vi "connect.vi"(8 "error in (no error)":errorcluster, 11 "TCPClient in":refnum<class "TCPClient.lvclass">) -> (0 "error out":errorcluster, 3 "TCPClient out":refnum<class "TCPClient.lvclass">)   [LabVIEW 2016, in "tcp.lvlib" / "TCPClient.lvclass"]
uses:
  TCPClient.lvclass
  TCPClient.lvclass/TCPClient.ctl
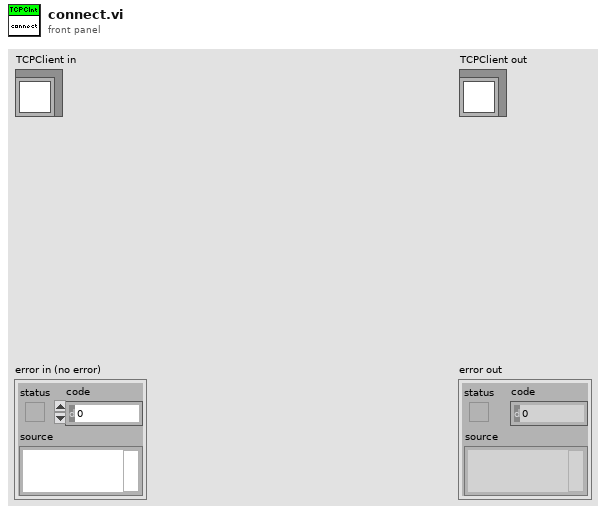
[diagram p1: front panel]
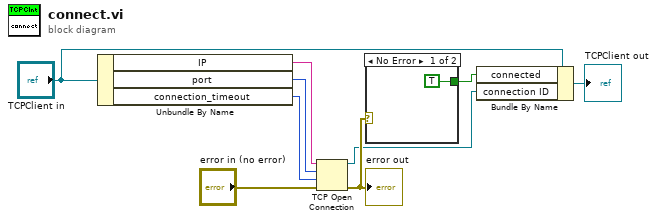
[diagram p0: block diagram]
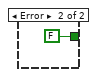
[diagram p2: hidden frame]
diagram:
  n1 = Unbundle By Name("TCPClient in") -> ("IP"=w3:string, "port"=w2:u16, "connection_timeout"=w1:i32)
  n2 = TCP Open Connection(address=w3, remote port or service name=w2, timeout ms (60000)=w1, error in (no error)="error in (no error)") -> (connection ID=w4:refnum<k5>, error out=w8:errorcluster)  [unwired: 1 in]
  "error out" <- w8
  n3 = case shown="No Error" w8 {
    tunnel: [TRUE ("connected") FALSE ("connected")] -> w5
    frame No Error {
    }
    frame Error {
    }
  }
  n4 = Bundle By Name(cluster="TCPClient in", "connected"=w5, "connection ID"=w4) -> (→"TCPClient out":refnum<class "TCPClient.lvclass">)
